vi "TPNT_OpenDeviceData.vi"(8 "error in (no error)":errorcluster, 10 "Name":string) -> (0 "error out":errorcluster, 3 "Data Refnum out":T1, 4 "Created New":bool)   [LabVIEW 2016]
uses:
  TPNT_Refnum.ctl
  TPNT_CoreFunction.ctl
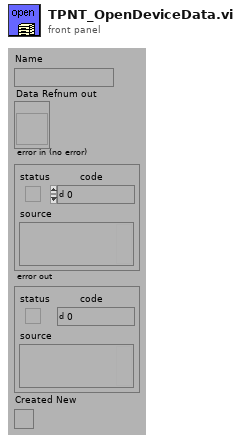
[diagram p1: front panel]
types:
  T1 = typedef "TPNT_Refnum.ctl" = refnum<vi>
  T2 = typedef "TPNT_CoreFunction.ctl" = enum16{"Reset", "Register", "Get Data", "Set Data", "Unregister", "Test", "Get Objects"}
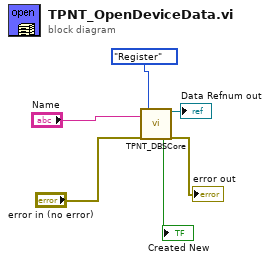
[diagram p0: block diagram]
diagram:
  n1 = call "TPNT_DBSCore.vi"("Name"="Name", "error in (no error)"="error in (no error)", "Function (Get Data)"=TPNT_CoreFunction."Register") -> ("Created New"=→"Created New":bool, "Object Refnum out"=→"Data Refnum out":T1, "error out"=→"error out":errorcluster)  [unwired: 2 in, 12 out]
